vi "TEST - Save VI ConPane Image.vi"(8 "error in (no error)":errorcluster) -> (0 "error out":errorcluster, 2 "pass":bool)   [LabVIEW 2020, in "test_openg_application_control.lvlib"]
uses:
  <userlib>/_OpenG.lib/file/file.llb/Convert File Extension (Path)__ogtk.vi
  test_openg_application_control.lvlib
  <userlib>/_OpenG.lib/error/error.llb/openg_error.lvlib
  source/library/openg_application_control.lvlib
  <userlib>/_OpenG.lib/file/file.llb/openg_file.lvlib
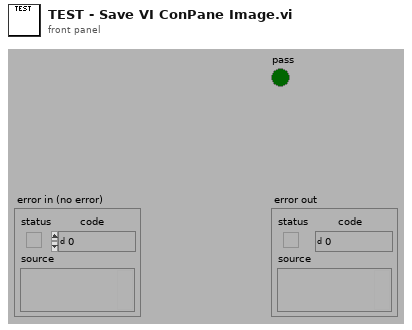
[diagram p1: front panel]
types:
  T1 = typedef "imagedata.ctl" = cluster{"image type":i32, "image depth":i32, "image":u8[], "mask":u8[], "colors":u32[], "Rectangle":cluster{"left":i16, "top":i16, "right":i16, "bottom":i16}}
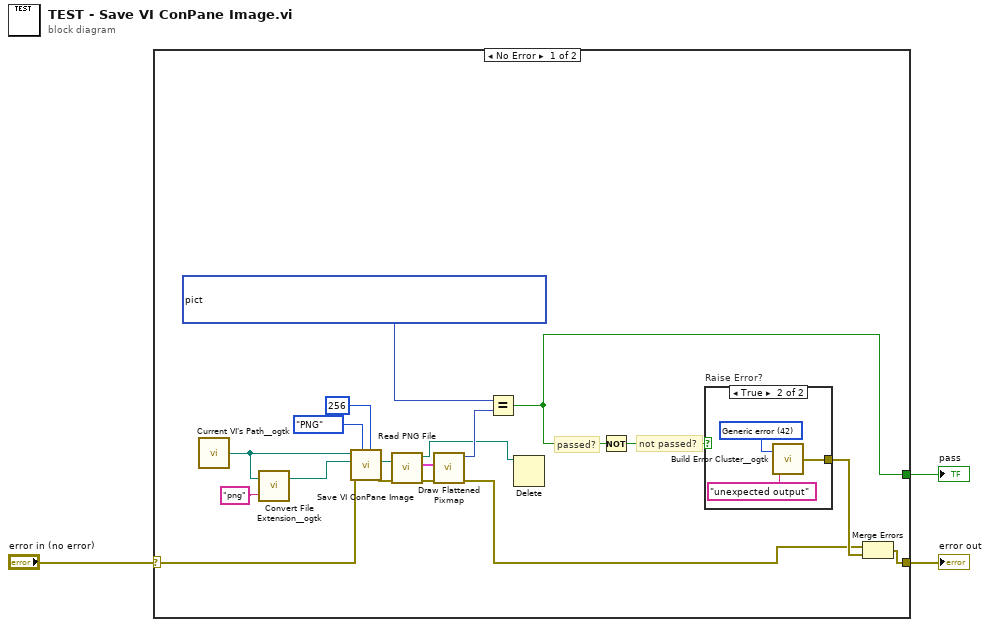
[diagram p0: block diagram]
diagram:
  n1 = case shown="No Error" "error in (no error)" {
    selector: "error in (no error)" -> [w12 w23]
    tunnel: [w11 _] -> w3
    tunnel: [w19 w23] -> w1
    frame No Error {
      # "not passed?"
      # "passed?"
      n2 = call <userlib>:"Current VI's Path__ogtk.vi"() -> ("Current VI's Path (+ Relative)"=w14:path)  [unwired: 1 in]
      n3 = call-poly <userlib>:"Convert File Extension__ogtk.vi"("new ending (none)"="png", "file name"=w14) -> ("new filename"=w9:path)  [unwired: 1 out]
      n4 = call "Save VI ConPane Image.vi"("Image Depth (256)"=256 ("Image Depth"), "Image Format"=enum32{"PNG", "JPEG", "GIF"}."PNG", "error in (no error)"=w12, "Image File Path"=w9, "VI Path"=w14) -> ("error out"=w6:errorcluster)  [unwired: 6 in]
      n5 = call <vilib>:"Read PNG File.vi"("error in (no error)"=w6, "path to PNG file"=w9) -> ("error out"=w7:errorcluster, "image data"=w10:T1, "path"=w5:path)  [unwired: 7 in]
      n6 = call <vilib>:"Draw Flattened Pixmap.vi"("image data"=w10) -> ("new picture"=w8:picture)  [unwired: 8 in]
      n7 = Equal?(x=picture bytes[13240] ("picture out"), y=w8) -> (x = y?=w11:bool)
      n8 = Delete(path (use dialog)=w5) -> ()  [unwired: 4 in, 3 out]
      n9 = Not(x=w11) -> (.not. x?=w17:bool)
      n10 = case "Raise Error?" shown="True" w17 {
        tunnel: [_ w20] -> w18
        frame False {
        }
        frame True {
          w21 = 42 items=["No error", "Argument error", "Memory is full", "Out of zone", "End of file", "File already open", "Generic file I/O error", "File not found", "File permission error", "Disk is full", "Duplicate path", "Too many files open", "System feature not enabled", "Resource file not found", "Cannot add resource", "Resource not found", "Image not found", "Image memory error", "Pen does not exist", "Config type invalid", "Config token not found", "Config parse error", "Config memory error", "Bad external code format", "Bad external code offset", "External code not present", "Null window", "Destroy window error", "Null menu", "Print aborted", "Bad print record", "Print driver error", "Windows error during printing", "Memory error during printing", "Print dialog error", "Generic print error", "Invalid device refnum", "Device not found", "Device parameter error", "Device unit error", "Cannot open device", "Device call aborted", "Generic error", "Cancelled by user", "Object ID too low", "Object ID too high", "Object not in heap", "Unknown heap", "Unknown object (invalid DefProc)", "Unknown object (DefProc not in table)", "Message out of range", "Invalid (null) method", "Unknown message", "Manager call not supported", "Bad address", "Network operation in progress", "Network operation timed out", "Connection is busy", "Network attribute not supported", "Network error", "Address in use", "System out of memory", "Connection aborted", "Connection refused", "Not connected", "Already connected", "Connection closed", "Initialization error (interapplication manager)", "Bad occurrence", "Wait on unbound occurrence handler", "Occurrence queue overflow", "Datalog type conflict", "Unused", "Unrecognized type (interapplication manager)", "Memory corrupt", "Failed to make temporary DLL", "Old CIN version", "Drag socket not found", "Failed to load drop-object", "Failed to register OLE object", "Failed to release OLE object", "Format specifier type mismatch", "Unknown format specifier", "Too few format specifiers", "Too many format specifiers", "Scan failed", "Newer CIN version", "Error converting to variant", "Runtime menu error", "Password tampered", "Variant attribute not found", "Incompatible variant data type", "Event data is not available", "Event Store is not present", "Occurrence is not found", "Event Queue is not created", "Event info is not available", "Refnum passed is NULL", "Error retrieving Class GUID", "Error retrieving CoClass GUID", "Error retrieving TypeLib GUID.", "Bad built application magic bytes.", "Specific driver is different from the specific driver associated with the Logical Name.", "There is no session opened to the class driver.", "Max Error", "MAX - Error with config objects", "MAX - Error loading configuration", "MAX - Group not supported"]
          n11 = call <userlib>:"Build Error Cluster__ogtk.vi"("String to Prepend to source (\"\")"="unexpected output" ("String to Prepend to source (\"\")"), "code"=w21) -> ("error out"=w20:errorcluster)
        }
      }
      n12 = Merge Errors(w7, w18) -> (w19:errorcluster)
    }
    frame Error {
    }
  }
  "pass" <- w3
  "error out" <- w1
